vi "CheckErrorCluster.vi"(9 "Value":variant) -> (4 "error cluster":bool)   [LabVIEW 2014, in "Raspberry Pi Compatible Compiler for LabVIEW.lvlib" / "Python Functions.lvlib"]
uses:
  Python Functions.lvlib
  <vilib>/Utility/VariantDataType/Type.ctl
  <vilib>/Utility/VariantDataType/VariantType.lvlib
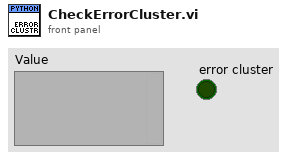
[diagram p1: front panel]
types:
  T1 = typedef "VariantType.lvlib/Type.ctl" = enum8{"Invalid Type", "Void", "I8", "I16", "I32", "I64", "U8", "U16", "U32", "U64", "Single Float", "Double Float", "Extended Float", "Single Complex", "Double Complex", "Extended Complex", "Enum U8", "Enum U16", "Enum U32", "Enum U64", "Single Float With Unit", "Double Float With Unit", "Extended Float With Unit", "Single Complex with Unit", "Double Complex with Unit", "Extended Complex with Unit", "Boolean", "String", "Path", "Picture", "Tag", "Array", "Cluster", "Variant", "LV Variant", "Waveform", "Timestamp", "Digital Waveform", "Digital Data", "ExpressData", "Refnum", "External Data", "VI", "Poly VI", "LabVIEW Class Instance", "Fixed Point"}
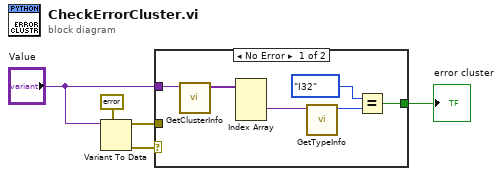
[diagram p0: block diagram]
diagram:
  n1 = Variant To Data(type=errorcluster {"status"=FALSE, "code"=0, "source"=""} ("error constant"), Variant="Value") -> (data=w3:errorcluster, error out=w4:errorcluster)  [unwired: 1 in]
  n2 = case shown="No Error" w4 {
    tunnel: "Value" -> [w11 _]
    tunnel: w3 -> [_ _]
    tunnel: [w6 _] -> w2
    frame No Error {
      n3 = call <vilib>:"GetClusterInfo.vi"("Variant"=w11) -> ("Cluster Elements"=w10:variant[])  [unwired: 9 in, 1 out]
      n4 = Index Array(array=w10) -> (element #2=w9:variant)  [unwired: 3 in, 2 out]
      n5 = call <vilib>:"GetTypeInfo.vi"("Variant"=w9) -> ("Type Enum"=w8:T1)  [unwired: 6 in, 4 out]
      n6 = Equal?(x=Type."I32", y=w8) -> (x = y?=w6:bool)
    }
    frame Error {
    }
  }
  "error cluster" <- w2
